vi "Convert Laser Intensity to Color.vi"(2 "Color Table":u32[](array[numeric])) -> (7 "Color Array":T1[](array[typedef]))   [LabVIEW 2017]
doc: "SubVI for Velodyne HDL-64E S2 Acquire and Graph - 3D.vi. Converts the LIDAR data to a color based on intensity."
uses:
  <vilib>/Utility/miscctls.llb/LVRGBAColorTypeDef.ctl
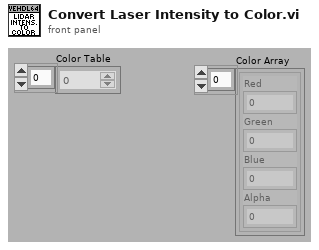
[diagram p1: front panel]
types:
  T1 = typedef "LVRGBAColorTypeDef.ctl" = cluster{"Red":sgl, "Green":sgl, "Blue":sgl, "Alpha":sgl}
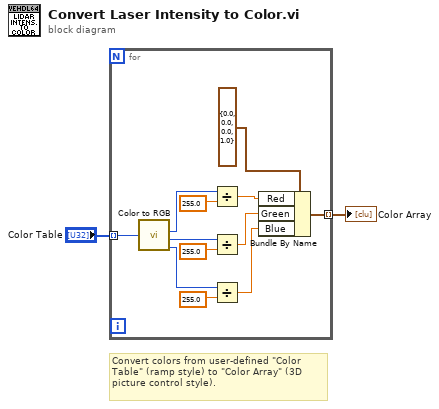
[diagram p0: block diagram]
diagram:
  # "Convert colors from user-defined \"Color Table\" (ramp style) to \"Color Array\" (3D picture control style)."
  n1 = for {
    tunnel: [w14] -> w2 mode=indexing
    tunnel: "Color Table" -> [w3] mode=indexing
    n2 = call <vilib>:"Color to RGB.vi"("Color"=w3) -> ("R"=w9:u8, "G"=w12:u8, "B"=w13:u8)  [unwired: 1 out]
    n3 = Divide(x=w9, y=sgl 255.0) -> (x/y=w6:sgl)
    n4 = Divide(x=w12, y=sgl 255.0) -> (x/y=w5:sgl)
    n5 = Divide(x=w13, y=sgl 255.0) -> (x/y=w4:sgl)
    n6 = Bundle By Name(cluster=T1 {"Red"=0.0, "Green"=0.0, "Blue"=0.0, "Alpha"=1.0} ("Color"), "Red"=w6, "Green"=w5, "Blue"=w4) -> (w14:T1)
  }
  "Color Array" <- w2
